vi "New Results (to override).vi"(7 "Image Nr.":i32, 8 "error in (no error)":errorcluster, 9 "Results In":refnum<class "Analyze Results Base.lvclass">[](array[class]), 10 "Parameters":refnum<class "Analyze Parameter Base.lvclass">[](array[class]), 11 "POLARIS Target Focus Actor In":refnum<class "POLARIS Target Focus Actor.lvclass">) -> (0 "error out":errorcluster, 3 "POLARIS Target Focus Actor Out":refnum<class "POLARIS Target Focus Actor.lvclass">)   [LabVIEW 2014, in "POLARIS Target Focus Actor.lvlib" / "POLARIS Target Focus Actor.lvclass"]
uses:
  POLARIS Target Focus Actor.lvclass
  Analyze/Results and Overlays/Results Base/Analyze Results Base.lvclass
  Analyze/Analyze Parameter/Analyze Parameter Base/Analyze Parameter Base.lvclass
  Analyze/Results and Overlays/Results q-Factor/Analyze Results q-Factor.lvclass
  Analyze/Results and Overlays/Results q-Factor/Analyze Results q-Factor.lvclass/Analyze Results q-Factor.ctl
  Analyze/Results and Overlays/Results q-Factor/Read q.vi
  Analyze/Results and Overlays/Results q-Factor/Read A.vi
  Applications/HIJ Vision Camera App/HIJ Vision Camera App/HIJ Vision Camera App.lvclass
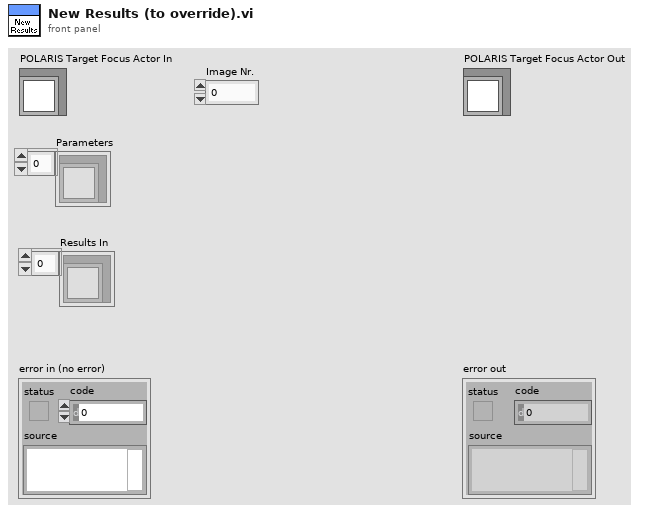
[diagram p1: front panel]
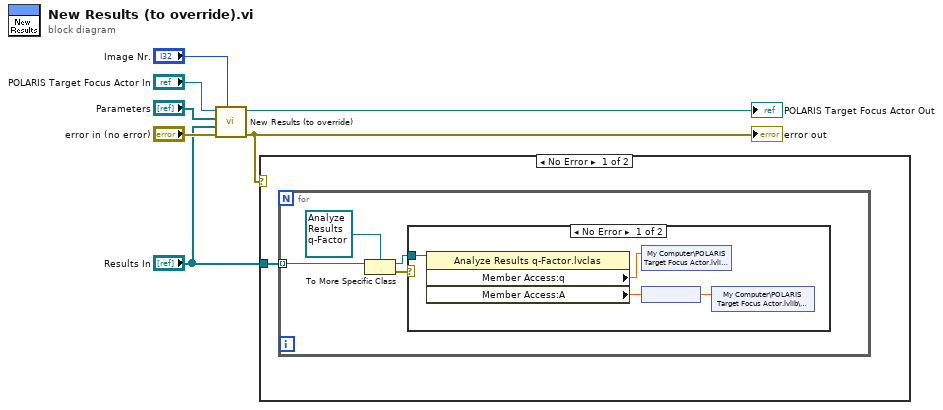
[diagram p0: block diagram]
diagram:
  n1 = call-parent "New Results (to override).vi"("Image Nr."="Image Nr.", "error in (no error)"="error in (no error)", "Results In"="Results In", "Parameters"="Parameters", "HIJ Vision Camera App In"="POLARIS Target Focus Actor In") -> ("error out"=w1:errorcluster, "HIJ Vision Camera App Out"=→"POLARIS Target Focus Actor Out":refnum<class "POLARIS Target Focus Actor.lvclass">)  [unwired: 5 in]
  "error out" <- w1
  n2 = case shown="No Error" w1 {
    tunnel: "Results In" -> [w8 _]
    frame No Error {
      n3 = for {
        tunnel: w8 -> [w12] mode=indexing
        n4 = To More Specific Class(target class=refnum<class "Analyze Results q-Factor.lvclass"> refnum ("Analyze Results q-Factor.lvclass"), reference=w12) -> (specific class reference=w10:refnum<class "Analyze Results q-Factor.lvclass">, error out=w9:errorcluster)  [unwired: 1 in]
        n5 = case shown="No Error" w9 {
          tunnel: w10 -> [w16 _]
          frame No Error {
            n6 = property class="Analyze Results q-Factor.lvclas"(reference=w16) -> ("Member Access:q"=w15:dbl, "Member Access:A"=w14:dbl[unit])  [unwired: 1 in, 2 out]
            n7 = shared-variable "My Computer\\POLARIS Target Focus Actor.lvlib\\q-Factor"(w15) -> ()  [unwired: 1 in, 1 out]
            n8 = node(w14) -> (w13:dbl)
            n9 = shared-variable "My Computer\\POLARIS Target Focus Actor.lvlib\\Focus Area"(w13) -> ()  [unwired: 1 in, 1 out]
          }
          frame Error {
          }
        }
      }
    }
    frame Error {
    }
  }
